vi "attribute_read_string_simple.vi"(5 "Repeated Capability":string, 7 "Attribute":T1={"Identifier"="", "Descriptive Name"="", "Data Type"=enum."Integer 32", "Command"="", "Access"=enum."Read/Write", "Range Table"="", "Read Callback"="", "Write Callback"="", "Supported Models"="", "Instrument Options"="", "Index"=0, "OPC Wait"=FALSE, "No Status Check"=FALSE, "Cache Only"=FALSE}, 8 "error in":errorcluster caption="error in (no error)", 10 "Direct Attribute ID (\"\")":string, 11 "VISA resource name":refnum<visa-resource-name>) -> (0 "error out":errorcluster, 2 "String out":string, 3 "VISA resource name out":refnum<visa-resource-name>)   [LabVIEW 2020, in "Rohde&Schwarz RTx Oscilloscopes.lvlib" / "rsidr_core.lvlib"]
uses:
  rsidr_core.lvlib
  type_Attribute.ctl
  type_Attribute_Data_Type.ctl
  type_ReadWriteAccess.ctl
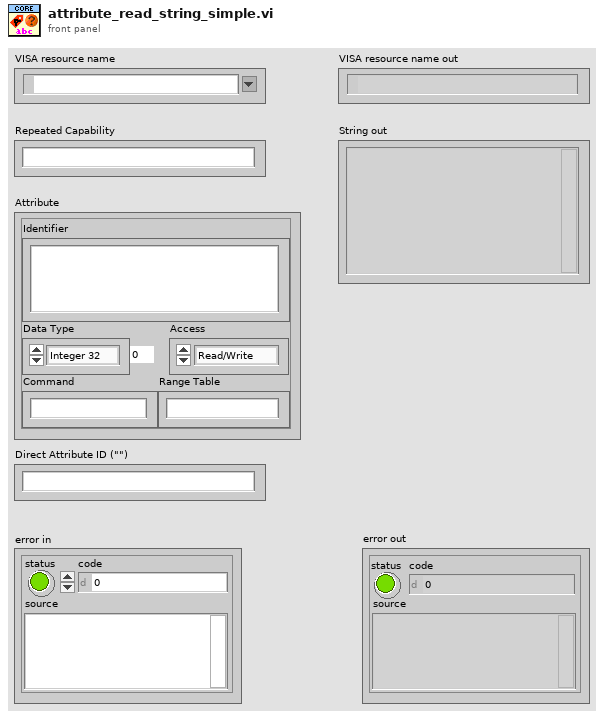
[diagram p1: front panel]
types:
  T1 = typedef "Rohde&Schwarz RTx Oscilloscopes.lvlib/rsidr_core.lvlib/type_Attribute.ctl" = cluster{"Identifier":string, "Descriptive Name":string, "Data Type":T2, "Command":string, "Access":T3, "Range Table":string, "Read Callback":string, "Write Callback":string, "Supported Models":string, "Instrument Options":string, "Index":i32, "OPC Wait":bool, "No Status Check":bool, "Cache Only":bool}
  T2 = typedef "Rohde&Schwarz RTx Oscilloscopes.lvlib/rsidr_core.lvlib/type_Attribute_Data_Type.ctl" = enum16{"Integer 32", "Double", "String", "Boolean", "None", "Integer 64", "RawString"}
  T3 = typedef "Rohde&Schwarz RTx Oscilloscopes.lvlib/rsidr_core.lvlib/type_ReadWriteAccess.ctl" = enum16{"Read Only", "Write Only", "Read/Write"}
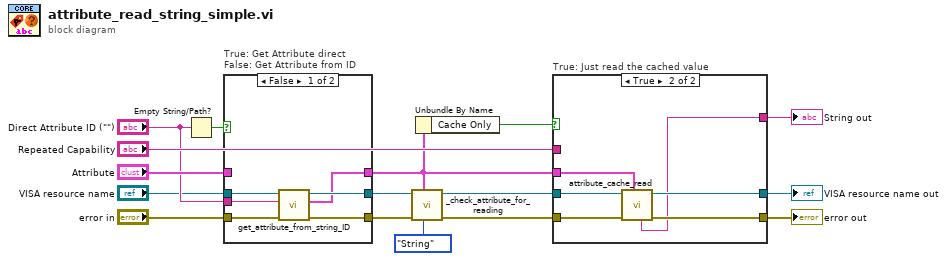
[diagram p0: block diagram]
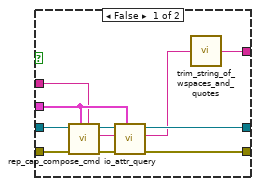
[diagram p3: hidden frame]
diagram:
  n1 = Empty String/Path?(string/path="Direct Attribute ID (\"\")") -> (empty?=w16:bool)
  n2 = case "True: Get Attribute direct\nFalse: Get Attribute from ID" shown="False" w16 {
    tunnel: "error in" -> [w22 w24]
    tunnel: [w20 w24] -> w7
    tunnel: "Direct Attribute ID (\"\")" -> [w18 _]
    tunnel: "Attribute" -> [_ w25]
    tunnel: [w17 w25] -> w2
    tunnel: "VISA resource name" -> [w21 w23]
    tunnel: [w19 w23] -> w6
    frame False {
      n3 = call "get_attribute_from_string_ID.vi"("error in"=w22, "Attribute ID in"=w18, "VISA resource name"=w21) -> ("error out"=w20:errorcluster, "Attribute out"=w17:T1, "VISA resource name out"=w19:refnum<visa-resource-name>)  [unwired: 6 in]
    }
    frame True {
    }
  }
  n4 = call "_check_attribute_for_reading.vi"("Expected Data Type"=type_Attribute_Data_Type."String", "Attribute"=w2, "error in"=w7, "VISA resource name"=w6) -> ("error out"=w5:errorcluster, "VISA resource name out"=w4:refnum<visa-resource-name>)  [unwired: 6 in]
  n5 = Unbundle By Name(w2) -> ("Cache Only"=w1:bool)
  n6 = case "True: Just read the cached value" shown="True" w1 {
    tunnel: "Repeated Capability" -> [w28 _]
    tunnel: [w31 w39] -> w9
    tunnel: [w30 w38] -> w10
    tunnel: [w26 w37] -> w11
    tunnel: w4 -> [w34 w41]
    tunnel: w5 -> [w35 w42]
    tunnel: w2 -> [w29 w40]
    frame False {
      n7 = call "rep_cap_compose_cmd.vi"("Repeated Capability"=w28, "Attribute"=w29, "error in"=w35, "VISA resource name"=w34) -> ("error out"=w33:errorcluster, "Command out"=w36:string, "VISA resource name out"=w32:refnum<visa-resource-name>)  [unwired: 5 in]
      n8 = call "io_attr_query.vi"("Attribute"=w29, "error in"=w33, "write buffer"=w36, "VISA resource name"=w32) -> ("error out"=w31:errorcluster, "read buffer"=w27:string, "VISA resource name out"=w30:refnum<visa-resource-name>)  [unwired: 5 in]
      n9 = call "trim_string_of_wspaces_and_quotes.vi"("String in"=w27) -> ("String out"=w26:string)  [unwired: 4 in]
    }
    frame True {
      n10 = call "attribute_cache_read.vi"("Attribute"=w40, "error in"=w42, "VISA resource name"=w41) -> ("error out"=w39:errorcluster, "VISA resource name out"=w38:refnum<visa-resource-name>, "String out"=w37:string)  [unwired: 1 in, 5 out]
    }
  }
  "error out" <- w9
  "VISA resource name out" <- w10
  "String out" <- w11
